vi "ToggleByRoomName.vi"(0 "reference in":refnum<class "MusicSystem.lvclass">, 2 "RoomName":string, 5 "Error In":errorcluster) -> (14 "reference out":refnum<class "MusicSystem.lvclass">, 19 "Error Out":errorcluster)   [LabVIEW 2024, in "MusicSystem.lvclass"]
uses:
  MusicSystem.lvclass
  House/Room_class/Room.lvclass
  MusicSystem.lvclass/MusicSystem.ctl
  Devices/MusicDevice_class/MusicDevice.lvclass
panel:
  # "Connector Pane"
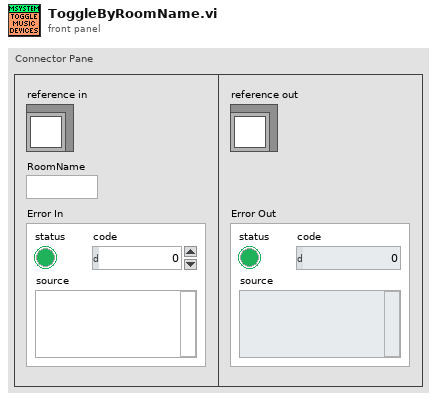
[diagram p1: front panel]
types:
  T1 = typedef "MusicSystem.lvclass/ObjectAttributes.ctl" = cluster{"Rooms":T2}
  T2 = typedef "Rooms Map.ctl" = map{string, refnum<class "Room.lvclass">}
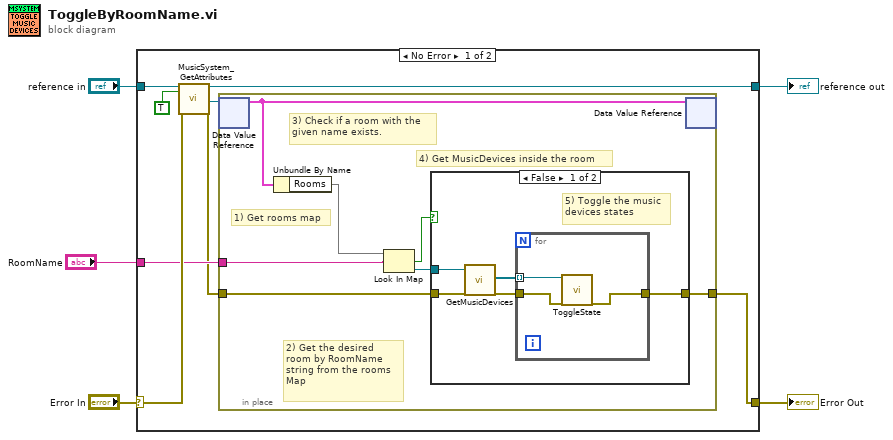
[diagram p0: block diagram]
diagram:
  n1 = case shown="No Error" "Error In" {
    selector: "Error In" -> [w12 w31]
    tunnel: [w6 w31] -> w4
    tunnel: [w11 w30] -> w2
    tunnel: "reference in" -> [w13 w30]
    tunnel: "RoomName" -> [w8 _]
    frame No Error {
      n2 = call "MusicSystem_GetAttributes.vi"("reference in"=w13, "OnlyGetDvrReference(False)"=TRUE, "Error In"=w12) -> ("reference out"=w11:refnum<class "MusicSystem.lvclass">, "DataRef"=w10:refnum<data-value>, "Error Out"=w7:errorcluster)  [unwired: 13 in, 1 out]
      n3 = in-place {
        in-place-border: w8 -> [w16]
        in-place-border: w7 -> [w15]
        in-place-border: [w14] -> w6
        # "4) Get MusicDevices inside the room"
        # "3) Check if a room with the\ngiven name exists."
        # "2) Get the desired\nroom by RoomName\nstring from the rooms\nMap"
        # "1) Get rooms map"
        n4 = in-place-dvr #1(w10) -> (w20:T1)  [unwired: 1 out]
        n5 = Unbundle By Name(w20) -> ("Rooms"=w17:T2)
        n6 = Look In Map(map=w17, key=w16) -> (key not found?=w19:bool, value=w18:refnum<class "Room.lvclass">)  [unwired: 1 in]
        n7 = case shown="False" w19 {
          tunnel: w18 -> [w25 _]
          tunnel: w15 -> [w22 w29]
          tunnel: [w21 w29] -> w14
          frame False {
            # "5) Toggle the music\ndevices states"
            n8 = call-dynamic "GetMusicDevices.vi"("reference in"=w25, "Error In"=w22) -> ("MusicDevices"=w24:refnum<class "MusicDevice.lvclass">[], "Error Out"=w23:errorcluster)  [unwired: 15 in, 1 out]
            n9 = for {
              tunnel: w24 -> [w26] mode=indexing
              tunnel: w23 -> [w28]
              tunnel: [w27] -> w21
              n10 = call "ToggleState.vi"("reference in"=w26, "Error In"=w28) -> ("Error Out"=w27:errorcluster)  [unwired: 16 in, 1 out]
            }
          }
          frame True {
          }
        }
        n11 = in-place-dvr #1(w20) -> ()  [unwired: 2 out]
      }
    }
    frame Error {
    }
  }
  "Error Out" <- w4
  "reference out" <- w2
